vi "Get All Operations.vi"(8 "error in (no error)":errorcluster caption="entrée d'erreur (pas d'erreur)", 11 "Operations en entrée":refnum<class "Operations.lvclass"> caption="DNL_LabVIEW Object in") -> (0 "error out":errorcluster caption="sortie d'erreur", 1 "Operations":T1[](array[typedef]), 2 "Keys":variant[](array[variant]), 3 "Operations en sortie":refnum<class "Operations.lvclass"> caption="DNL_LabVIEW Object out", 4 "tableau a afficher":string[][](array[string]))   [LabVIEW 2012, in "Operations.lvclass"]
uses:
  Operations.lvclass
  Operation/Operation Parameters.ctl
  Operation/Operation Type Enum.ctl
  controls/Currencies.ctl
  Operations.lvclass/Operations.ctl
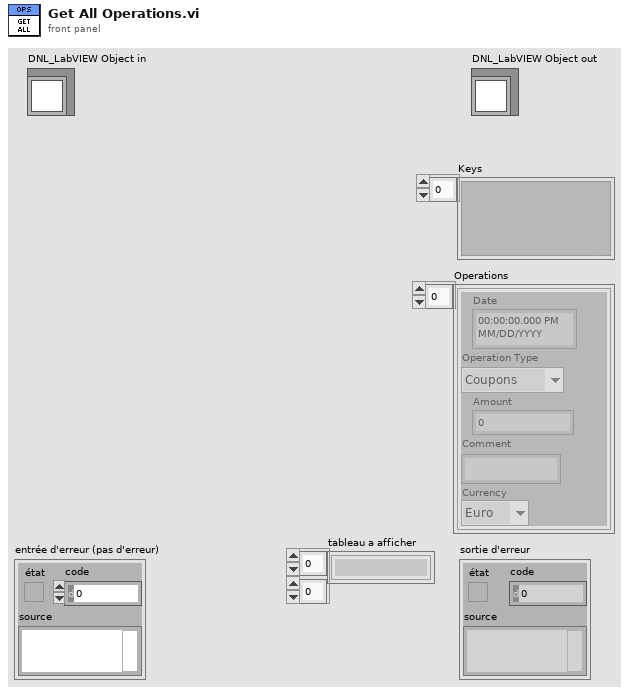
[diagram p1: front panel]
types:
  T1 = typedef "Operation Parameters.ctl" = cluster{"Date":timestamp, "Operation Type":T2, "Amount":dbl, "Comment":string, "Currency":T3}
  T2 = typedef "Operation Type Enum.ctl" = enum16{"Coupons", "Dépot", "Retrait", "Intérêts", "Taxe"}
  T3 = typedef "Currencies.ctl" = enum16{"Euro", "Dollar", "Yen", "RIM", "CHF"}
  T4 = typedef "Dictionary Object RefNum__ogtk.ctl" = refnum<k1>
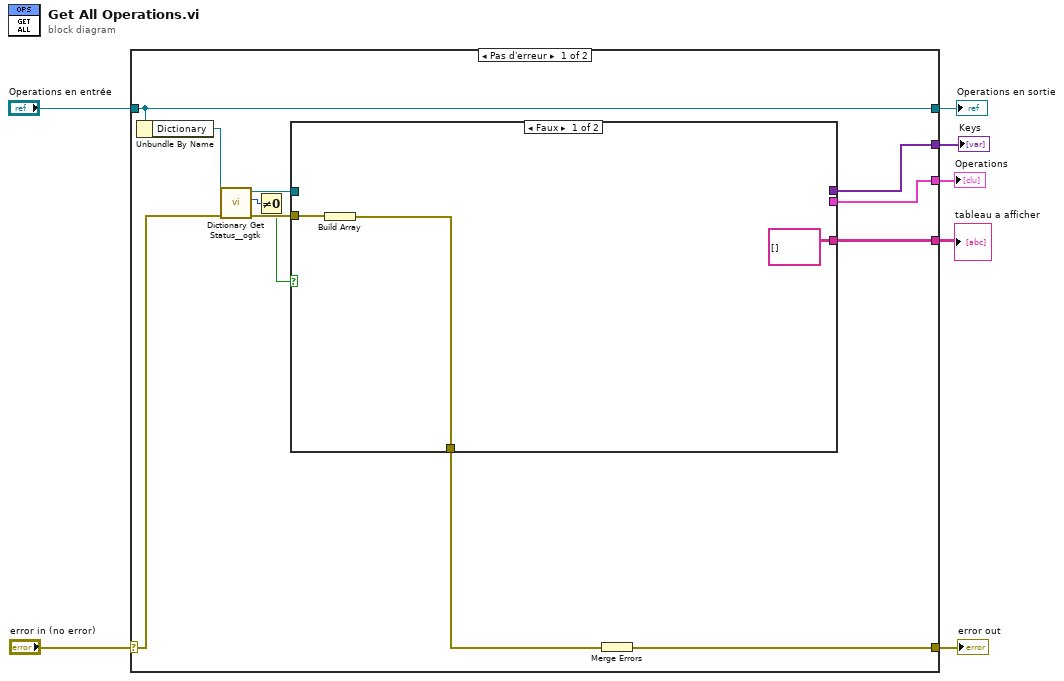
[diagram p0: block diagram]
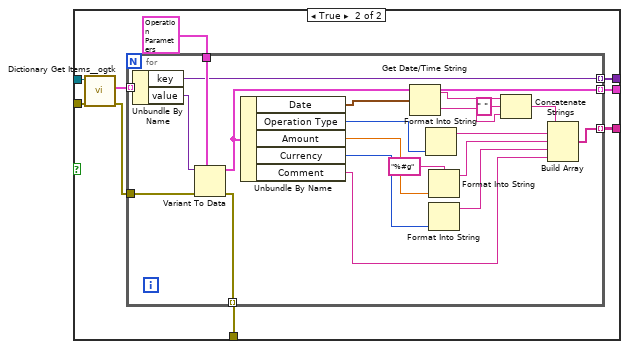
[diagram p2: hidden frame]
diagram:
  n1 = case shown="Pas d'erreur" "error in (no error)" {
    selector: "error in (no error)" -> [w12 w54]
    tunnel: [w17 w54] -> w6
    tunnel: [w19 w53] -> w4
    tunnel: "Operations en entrée" -> [w19 w53]
    tunnel: [w16 _] -> w3
    tunnel: [w15 _] -> w2
    tunnel: [w14 _] -> w1
    frame No Error {
      n2 = Unbundle By Name(w19) -> ("Dictionary"=w13:T4)
      n3 = call <userlib>:"Dictionary Get Status__ogtk.vi"("error in (no error)"=w12, "dictionary"=w13) -> ("error out"=w10:errorcluster, "size"=w9:i32, "dictionary out"=w11:T4)  [unwired: 7 in]
      n4 = Not Equal To 0?(x=w9) -> (x != 0?=w8:bool)
      n5 = case shown="Faux" w8 {
        tunnel: w11 -> [_ w31]
        tunnel: w10 -> [w21 w30]
        tunnel: [w20 w26] -> w18
        tunnel: [_ w25] -> w16
        tunnel: [_ w24] -> w15
        tunnel: [string[][] [] w23] -> w14
        frame False {
          n6 = Build Array(w21) -> (w20:errorcluster[])
        }
        frame True {
          n7 = call <userlib>:"Dictionary Get Items__ogtk.vi"("error in (no error)"=w30, "dictionary"=w31) -> ("error out"=w27:errorcluster, "items"=w29:cluster{"key":variant, "value":variant}[])  [unwired: 7 in, 1 out]
          n8 = for {
            tunnel: w29 -> [w52] mode=indexing
            tunnel: T1 {"Date"=timestamp(0 s since 1904-01-01), "Operation Type"=enum."Coupons", "Amount"=0.0, "Comment"="", "Currency"=enum."Euro"} ("Parameters") -> [w51]
            tunnel: w27 -> [w49]
            tunnel: [w48] -> w26 mode=indexing
            tunnel: [w46] -> w25 mode=indexing
            tunnel: [w47] -> w24 mode=indexing
            tunnel: [w35] -> w23 mode=indexing
            n9 = Unbundle By Name(w52) -> ("key"=w47:variant, "value"=w50:variant)
            n10 = Variant To Data(error in=w49, type=w51, Variant=w50) -> (data=w46:T1, error out=w48:errorcluster)
            n11 = Unbundle By Name(w46) -> ("Date"=w45:timestamp, "Operation Type"=w42:T2, "Amount"=w40:dbl, "Currency"=w39:T3, "Comment"=w36:string)
            n12 = Get Date/Time String(seconds (now)=w45) -> (date string=w44:string, time string=w32:string)  [unwired: 2 in]
            n13 = Format Into String(w42) -> (resulting string=w41:string)  [unwired: 3 in, 1 out]
            n14 = Format Into String(format string="%#g" ("chaîne de format"), w40) -> (resulting string=w38:string)  [unwired: 2 in, 1 out]
            n15 = Format Into String(w39) -> (resulting string=w37:string)  [unwired: 3 in, 1 out]
            n16 = Concatenate Strings(w44, " " ("chaîne"), w32) -> (w43:string)
            n17 = Build Array(w43, w41, w38, w37, w36) -> (w35:string[])
          }
        }
      }
      n18 = Merge Errors(w18) -> (w17:errorcluster)
    }
    frame Error {
    }
  }
  "error out" <- w6
  "Operations en sortie" <- w4
  "Operations" <- w3
  "Keys" <- w2
  "tableau a afficher" <- w1
